vi "set poisition.vi"(4 "Mode":u16(ring) items=["Move to position", "Move to limit", "Redefine current position"], 5 "config":refnum<queue>, 6 "Slow down code\ndefault = 0":T1(ring), 7 "Position (deg)":dbl, 8 "error in (no error)":errorcluster, 9 "Instrument Ref In":refnum<k24>) -> (2 "error out":errorcluster, 3 "Instrument Ref Out":refnum<k24>)   [LabVIEW 2019, in "SubVI.lvlib"]
uses:
  SubVI.lvlib
  lib/QDInstrument.dll
  config.ctl
  Instrument.ctl
  <vilib>/NI/Modbus Library/API/Master/Modbus Master.lvclass
panel:
  # "(真是通道1，假是通道2)"
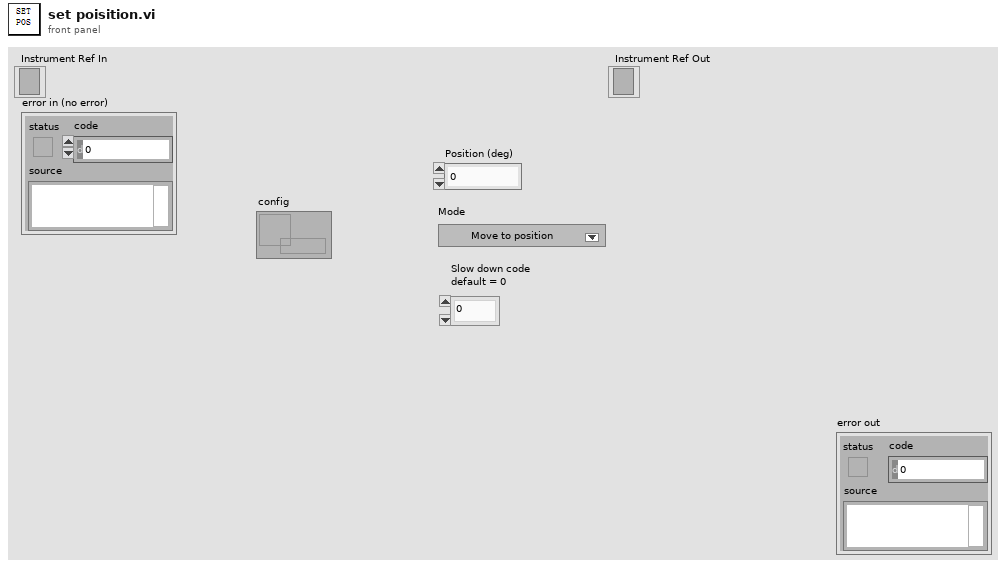
[diagram p1: front panel]
types:
  T1 = enum16{"0", "1", "2", "3", "4", "5", "6", "7", "8", "9", "10", "11", "12", "13", "14"}
  T2 = typedef "config.ctl" = cluster{"initialize":string, "6221":cluster{"6221 Resource":refnum<visa-resource-name>, "Delta status":bool}, "7001":cluster{"Ch":bool}, "SR830+6221":cluster{"source":u16, "阻抗":dbl, "量程入 4":i32, "量程入 3":i32, "量程入 2":i32, "量程入 1":i32, "电流":dbl, "SR830 2":bool, "SR830 3":bool, "SR830 4":bool, "SR830 1":bool, "VISA 1":refnum<visa-resource-name>, "VISA 2":refnum<visa-resource-name>, "VISA 3":refnum<visa-resource-name>, "VISA 4":refnum<visa-resource-name>, "量程":enum16{"量程每次测量会判定", "量程不变为设定值"}}, "2400":cluster{"2400":bool, "VISA":refnum<visa-resource-name>}, "ch":cluster{"ch str":string, "ch1":bool, "ch2":bool, "布尔":bool}, "error":bool, "数据文件路径":path, "log":cluster{"log路径":path, "log interval":dbl}, "Instrument":T3}
  T3 = typedef "Instrument.ctl" = cluster{"335 Resource":refnum<visa-resource-name>, "Input (0:A)":u16, "Instrument Type":i32, "quantum design":refnum<k24>, "Heater Output (1:1)":u16, "335state":refnum<vi>, "semaphore":T4, "TCP master instance":refnum<class "Modbus Master.lvclass">}
  T4 = typedef "Semaphore RefNum" = refnum<k1>
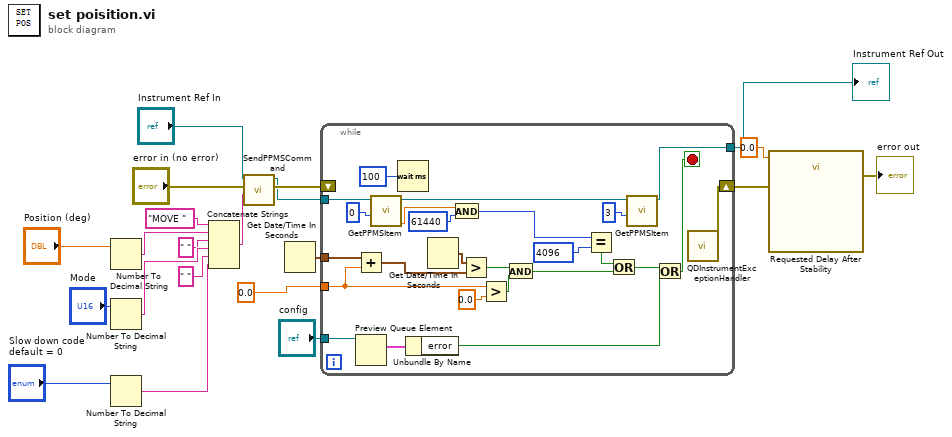
[diagram p0: block diagram]
diagram:
  n1 = Number To Decimal String(number="Position (deg)") -> (decimal integer string=w10:string)  [unwired: 1 in]
  n2 = Number To Decimal String(number="Mode") -> (decimal integer string=w13:string)  [unwired: 1 in]
  n3 = Number To Decimal String(number="Slow down code\ndefault = 0") -> (decimal integer string=w16:string)  [unwired: 1 in]
  n4 = Concatenate Strings("MOVE " ("string"), w10, " " ("string"), w13, " " ("string"), w16) -> (w17:string)
  n5 = call "SendPPMSCommand.vi"("PpmsCommand"=w17, "error in (no error)"="error in (no error)", "Instrument Ref In"="Instrument Ref In") -> ("error out"=w21:errorcluster, "Instrument Ref Out"=w20:refnum<k24>)  [unwired: 4 in, 3 out]
  n6 = Get Date/Time In Seconds() -> (seconds since 1Jan1904=w19:timestamp)
  n7 = while {
    shift-right: [w37] -> w18
    shift-left: w21 -> [_]
    tunnel: w19 -> [w45]
    tunnel: 0.0 ("Timeout") -> [w42]
    tunnel: w20 -> [w36]
    tunnel: [w27] -> w6
    tunnel: "config" -> [w26]
    stop <- w24 stop-if-true
    n8 = Add(x=w45, y=w42) -> (x+y=w43:timestamp)
    n9 = Preview Queue Element(queue=w26) -> (element=w23:T2)  [unwired: 2 in, 3 out]
    n10 = call "GetPPMSItem.vi"("Channel"=0, "Instrument Ref In"=w36) -> ("Result"=w30:dbl, "Instrument Ref Out"=w28:refnum<k24>)  [unwired: 2 in, 2 out]
    n11 = Wait (ms)(milliseconds to wait=u32 100) -> ()  [unwired: 1 out]
    n12 = Unbundle By Name(w23) -> ("error"=w22:bool)
    n13 = Get Date/Time In Seconds() -> (seconds since 1Jan1904=w44:timestamp)
    n14 = And(x=w30, y=61440) -> (x .and. y?=w34:i32)
    n15 = Greater?(x=w44, y=w43) -> (0:w40:bool)
    n16 = Greater?(x=w42, y=0.0) -> (0:w39:bool)
    n17 = And(x=w40, y=w39) -> (x .and. y?=w38:bool)
    n18 = Equal?(x=w34, y=4096) -> (x = y?=w32:bool)
    n19 = Or(x=w32, y=w38) -> (x .or. y?=w25:bool)
    n20 = call "GetPPMSItem.vi"("Channel"=3, "Instrument Ref In"=w28) -> ("Instrument Ref Out"=w27:refnum<k24>)  [unwired: 2 in, 3 out]
    n21 = Or(x=w25, y=w22) -> (x .or. y?=w24:bool)
    n22 = call "QDInstrumentExceptionHandler.vi"() -> ("Error out"=w37:errorcluster)  [unwired: 1 in]
  }
  "Instrument Ref Out" <- w6
  n23 = call "Requested Delay After Stability"("error in (no error)"=w18, "Delay Time (s)"=0.0) -> ("error out"=→"error out":errorcluster)  [unwired: 9 in]
